vi "Climb Controller Interactive Check.vi"(8 "Interactive Command in":T1={"Operation"=enum."Reserve", "Setpoint"=0.0, "Duration"=0.0, "Climb States"=enum."Deploy"}, 9 "Default Command":T1={"Operation"=enum."Reserve", "Setpoint"=0.0, "Duration"=0.0, "Climb States"=enum."Deploy"}, 11 "Buttons":cluster{"Execute Cmd":bool, "Abort Cmd":bool}) -> (1 "Interactive Command out":T1={"Operation"=enum."Reserve", "Setpoint"=0.0, "Duration"=0.0, "Climb States"=enum."Deploy"}, 2 "Trace String":string, 3 "Schedule":bool)   [LabVIEW 2023]
doc: "Check the Execute and Abort buttons and choose the data and trace string."
uses:
  Climb Setpoints.ctl
  Climb Operations.ctl
  Support Code/Teleop Util/Climb States.ctl
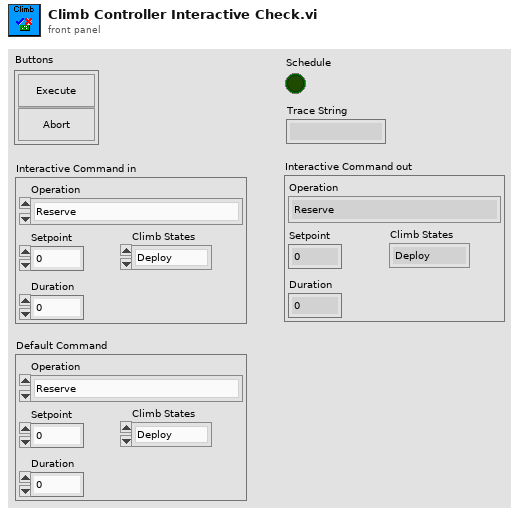
[diagram p1: front panel]
types:
  T1 = typedef "Climb Setpoints.ctl" = cluster{"Operation":T2, "Setpoint":dbl, "Duration":dbl, "Climb States":T3}
  T2 = typedef "Climb Operations.ctl" = enum16{"Reserve", "Read Current", "Immediate"}
  T3 = typedef "Climb States.ctl" = enum16{"Idle", "Deploy", "Undeploy", "Manual Overrides"}
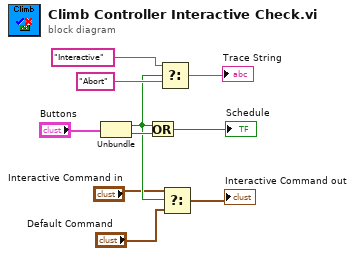
[diagram p0: block diagram]
diagram:
  n1 = Unbundle("Buttons") -> ("Execute Cmd"=w6:bool, "Abort Cmd"=w7:bool)
  n2 = Or(x=w6, y=w7) -> (x .or. y?=→"Schedule":bool)
  n3 = Select(t="Interactive", s=w6, f="Abort") -> (s? t:f=→"Trace String":string)
  n4 = Select(t="Interactive Command in", s=w6, f="Default Command") -> (s? t:f=→"Interactive Command out":T1)
